vi "Top App Check.vi"() -> ()   [LabVIEW 2018]
panel:
  out "Args":string[](array[string])
  out "Action":string
  out "CmdLine":bool
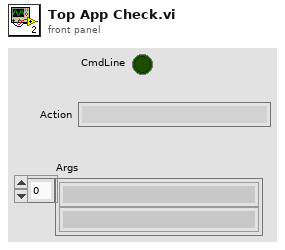
[diagram p1: front panel]
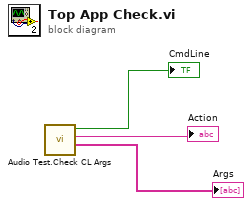
[diagram p0: block diagram]
diagram:
  n1 = call "Audio Test.Check CL Args.vi"() -> ("Args"=→"Args":string[], "Action"=→"Action":string, "CmdLine"=→"CmdLine":bool)  [unwired: 9 in]
